vi "contains.vi"(0 "reference":refnum<class "RectangularNode.lvclass">, 1 "point2D":T1 {"y" format="%.2f"; "x" format="%.2f"}, 2 "AdditionalMargin":i32, 5 "error in (no error)":errorcluster) -> (14 "reference out":refnum<class "RectangularNode.lvclass">, 15 "contains":bool, 19 "error out":errorcluster)   [LabVIEW 2016, in "RectangularNode.lvclass"]
doc: "contains"
uses:
  <resource>/Framework/Providers/Open_GDS/UML/RectangularNode_class/RectangularNode.lvclass
  C:/Program Files (x86)/National Instruments/LabVIEW 2016/resource/Framework/Providers/Open_GDS/UML/AbstractNode_class/AbstractNode.lvclass
  <resource>/Framework/Providers/Open_GDS/UML/General/Point/Point Point2D.ctl
  <resource>/Framework/Providers/Open_GDS/UML/AbstractNode_class/AbstractNode.lvclass
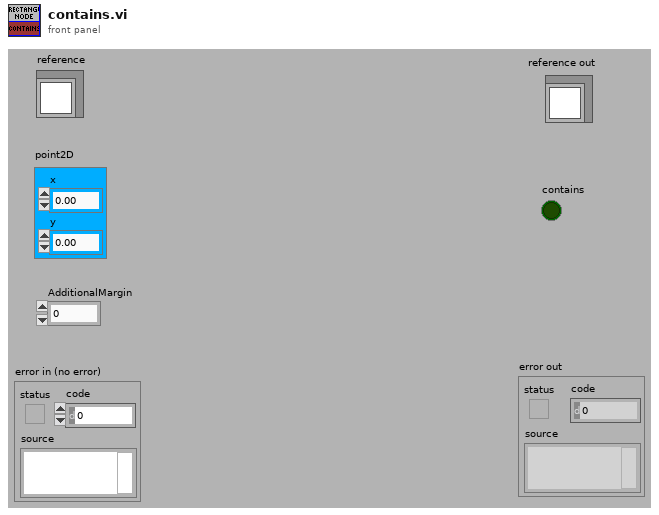
[diagram p1: front panel]
types:
  T1 = typedef "Point Point2D.ctl" = cluster{"x":dbl, "y":dbl}
  T2 = typedef "RectangularNode.lvclass/ObjectAttributes.ctl" = cluster{"bounds":T3}
  T3 = typedef "Rectangle Rectangle2D.ctl" = cluster{"x":dbl, "y":dbl, "width":dbl, "height":dbl}
  T4 = typedef "AbstractNode.lvclass/ObjectAttributes.ctl" = cluster{"parent":refnum<class "AbstractNode.lvclass">, "children":refnum<class "AbstractNode.lvclass">[], "Hidden":bool}
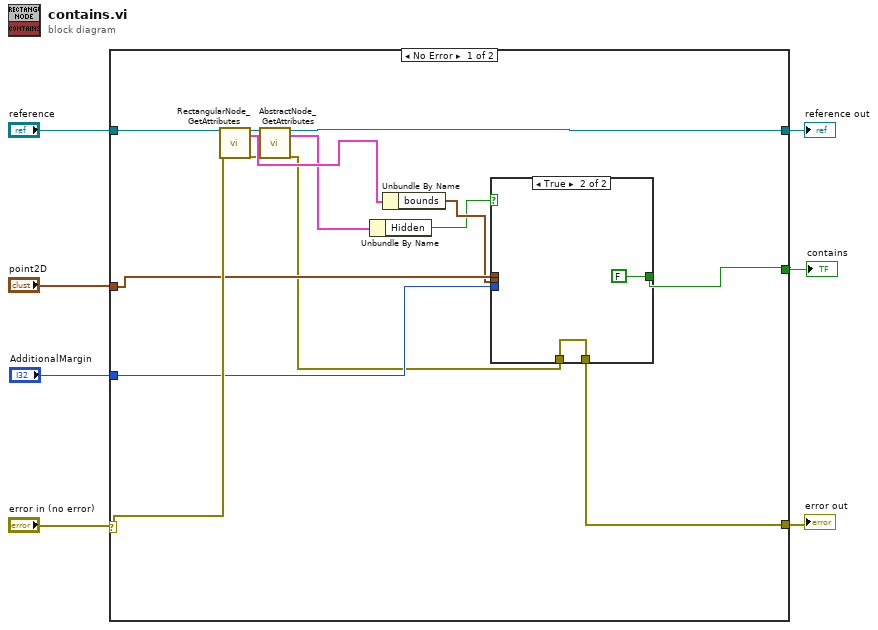
[diagram p0: block diagram]
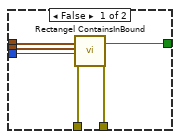
[diagram p2: hidden frame]
diagram:
  n1 = case shown="No Error" "error in (no error)" {
    selector: "error in (no error)" -> [w19 w30]
    tunnel: "reference" -> [w21 w31]
    tunnel: [w20 w30] -> w6
    tunnel: [w9 w31] -> w5
    tunnel: "point2D" -> [w18 _]
    tunnel: [w17 _] -> w2
    tunnel: "AdditionalMargin" -> [w15 _]
    frame No Error {
      n2 = call <resource>:"RectangularNode_GetAttributes.vi"("reference in"=w21, "error in (no error)"=w19) -> ("reference out"=w12:refnum<class "RectangularNode.lvclass">, "Data"=w13:T2, "error out"=w11:errorcluster)  [unwired: 1 in, 14 out]
      n3 = call <resource>:"AbstractNode_GetAttributes.vi"("reference in"=w12, "error in (no error)"=w11) -> ("reference out"=w9:refnum<class "RectangularNode.lvclass">, "Data"=w8:T4, "error out"=w10:errorcluster)  [unwired: 14 in, 1 out]
      n4 = Unbundle By Name(w8) -> ("Hidden"=w14:bool)
      n5 = Unbundle By Name(w13) -> ("bounds"=w16:T3)
      n6 = case shown="True" w14 {
        tunnel: [w27 w29] -> w20
        tunnel: w18 -> [w26 _]
        tunnel: [w25 FALSE ("contains")] -> w17
        tunnel: w16 -> [w24 _]
        tunnel: w10 -> [w23 w29]
        tunnel: w15 -> [w22 _]
        frame False {
          n7 = call <resource>:"Rectangel ContainsInBound.vi"("point2D"=w26, "bounds"=w24, "AdditionalMargin"=w22, "error in (no error)"=w23) -> ("contains"=w25:bool, "error out"=w27:errorcluster)  [unwired: 14 out]
        }
        frame True {
        }
      }
    }
    frame Error {
    }
  }
  "reference out" <- w5
  "error out" <- w6
  "contains" <- w2
